vi "createEventForceActuatorSafetyChecks.vi"(8 "error in (no error)":errorcluster, 11 "UserEvents in":refnum<class "UserEvents.lvclass">) -> (0 "error out":errorcluster, 3 "UserEvents out":refnum<class "UserEvents.lvclass">)   [LabVIEW 2016, in "UserEvents.lvclass"]
uses:
  UserEvents.lvclass
  DataTypes/Topics/EventForceActuatorSafetyChecks.ctl
  DataTypes/Topics/Parts/Timestamp.ctl
  UserEvents.lvclass/UserEvents.ctl
  DataTypes/Topics/M1M3SupportTopics.lvlib
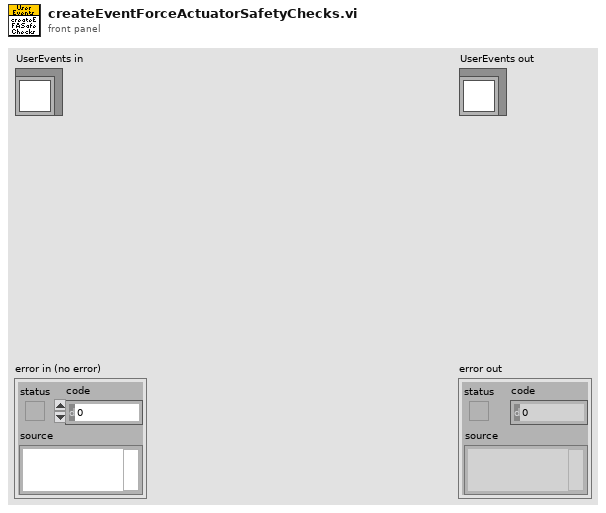
[diagram p1: front panel]
types:
  T1 = typedef "M1M3SupportTopics.lvlib/EventForceActuatorSafetyChecks.ctl" = cluster{"Timestamp":T2, "AllInSafetyLimit":bool, "SafetyLimitOk":bool[], "MirrorWeightOk":bool, "XMomentOk":bool, "YMomentOk":bool, "AllNeighborsOk":bool, "NeighborsOk":bool[], "MagnitudeOk":bool, "AllGlobalBendingOk":bool, "GlobalBendingOk":bool[], "FollowingErrorOk":bool, "AxialFollowingErrorOk":bool[], "LateralFollowingErrorOk":bool[], "AOSNetForceOk":bool, "AllElevationForcesOk":bool, "ElevationForcesOk":bool[], "AllAzimuthForcesOk":bool, "AzimuthForcesOk":bool[], "AllThermalForcesOk":bool, "ThermalForcesOk":bool[], "AllAOSForcesOk":bool, "AOSForcesOk":bool[]}
  T2 = typedef "M1M3SupportTopics.lvlib/Timestamp.ctl" = dbl
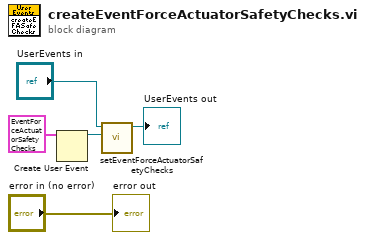
[diagram p0: block diagram]
diagram:
  n1 = Create User Event(user event datatype=T1 {"Timestamp"=0.0, "AllInSafetyLimit"=FALSE, "SafetyLimitOk"=[], "MirrorWeightOk"=FALSE, "XMomentOk"=FALSE, "YMomentOk"=FALSE, "AllNeighborsOk"=FALSE, "NeighborsOk"=[], "MagnitudeOk"=FALSE, "AllGlobalBendingOk"=FALSE, "GlobalBendingOk"=[], "FollowingErrorOk"=FALSE, "AxialFollowingErrorOk"=[], "LateralFollowingErrorOk"=[], "AOSNetForceOk"=FALSE, "AllElevationForcesOk"=FALSE, "ElevationForcesOk"=[], "AllAzimuthForcesOk"=FALSE, "AzimuthForcesOk"=[], "AllThermalForcesOk"=FALSE, "ThermalForcesOk"=[], "AllAOSForcesOk"=FALSE, "AOSForcesOk"=[]} ("EventForceActuatorSafetyChecks")) -> (user event=w3:refnum<user-event>)  [unwired: 1 in, 1 out]
  n2 = call "setEventForceActuatorSafetyChecks.vi"("EventForceActuatorSafetyChecks"=w3, "UserEvents in"="UserEvents in") -> ("UserEvents out"=→"UserEvents out":refnum<class "UserEvents.lvclass">)  [unwired: 9 in]
  "error out" <- "error in (no error)"
